vi "Dequeue Message.vi"(8 "error in (no error)":errorcluster, 11 "Message Queue":refnum<queue>) -> (0 "error out":errorcluster, 1 "Message Data":variant, 2 "Message":string, 3 "dup Message Queue":refnum<queue>)   [LabVIEW 2025, in "Message Queue.lvlib"]
doc: "This VI pulls messages off the Message Queue."
uses:
  Message Queue.lvlib
  Message Cluster.ctl
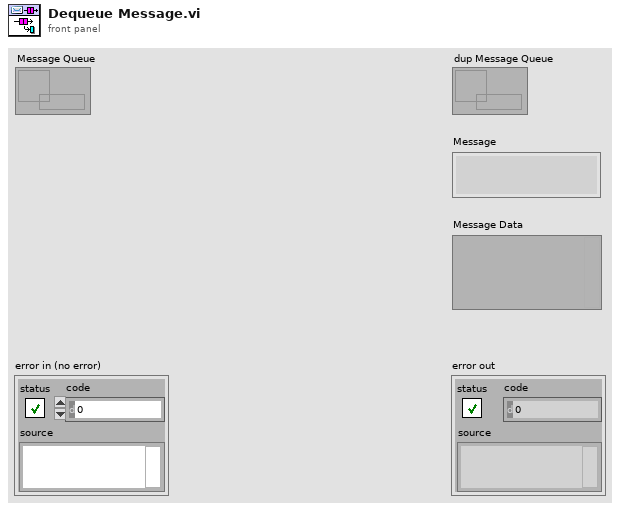
[diagram p1: front panel]
types:
  T1 = typedef "Message Queue.lvlib/Message Cluster.ctl" = cluster{"Message":string, "Message Data":variant}
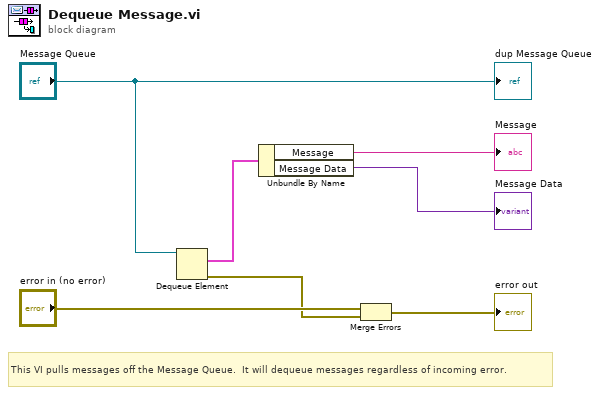
[diagram p0: block diagram]
diagram:
  # "This VI pulls messages off the Message Queue.  It will dequeue messages regardless of incoming error."
  n1 = Dequeue Element(queue="Message Queue") -> (element=w4:T1, error out=w1:errorcluster)  [unwired: 2 in, 2 out]
  n2 = Unbundle By Name(w4) -> ("Message"=→"Message":string, "Message Data"=→"Message Data":variant)
  n3 = Merge Errors("error in (no error)", w1) -> (→"error out":errorcluster)
  "dup Message Queue" <- "Message Queue"
